vi "PH_Synchrolock_Watch.Investigeate Trace.vi"(0 "Threshold":dbl, 1 "Width":i32, 2 "X Increment":dbl, 3 "Waveform Array":dbl[](array[numeric]), 5 "error in":errorcluster) -> (14 "Mean Amplitude":dbl, 15 "Peak Locations":dbl[](array[numeric]), 19 "error out":errorcluster)   [LabVIEW 2014, in "PH_Synchrolock_Watch.lvlib"]
doc: "This VI scales the incoming waveform, detects the pek position(s) and further information."
uses:
  PH_Synchrolock_Watch.lvlib
  <vilib>/Analysis/baseanly.llb/Mean (DBL).vi
  <vilib>/measure/mamon.llb/Waveform Peak Detection for 1 Chan.vi
  <vilib>/measure/NI_MAPro.lvlib
  <vilib>/Analysis/NI_AALBase.lvlib
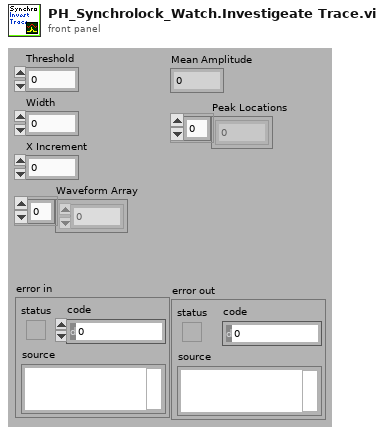
[diagram p1: front panel]
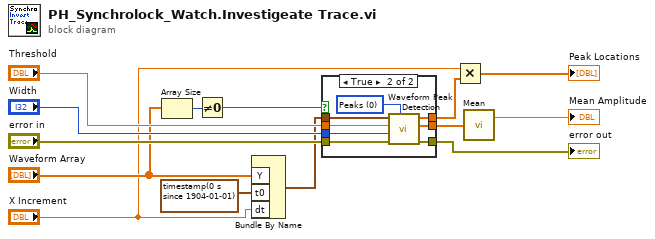
[diagram p0: block diagram]
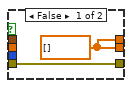
[diagram p2: hidden frame]
diagram:
  n1 = Array Size(array="Waveform Array") -> (size(s)=w9:i32)
  n2 = Not Equal To 0?(x=w9) -> (x != 0?=w8:bool)
  n3 = Bundle By Name("Y"="Waveform Array", "t0"=timestamp(0 s since 1904-01-01), "dt"="X Increment") -> (w7:waveform(dbl))  [unwired: 1 out]
  n4 = case shown="True" w8 {
    tunnel: "Threshold" -> [_ w24]
    tunnel: [w16 w23] -> w5
    tunnel: w7 -> [_ w22]
    tunnel: [w16 w21] -> w2
    tunnel: "Width" -> [_ w20]
    tunnel: "error in" -> [w15 w19]
    tunnel: [w15 w18] -> w14
    frame False {
      w16 = dbl[] [] ("Locations")
    }
    frame True {
      w17 = u16 0 items=["Peaks", "Valleys"] ("peaks/valleys")
      n5 = call-poly <vilib>:"Waveform Peak Detection.vi"("peaks/valleys"=w17, "error in"=w19, "width"=w20, "threshold"=w24, "Signal In"=w22) -> ("error out"=w18:errorcluster, "Amplitudes"=w21:dbl[], "Locations"=w23:dbl[])  [unwired: 2 in, 2 out]
    }
  }
  "error out" <- w14
  n6 = Multiply(x="X Increment", y=w5) -> (x*y=→"Peak Locations":dbl[])
  n7 = call-poly <vilib>:"Mean.vi"("X"=w2) -> ("mean"=→"Mean Amplitude":dbl)  [unwired: 1 out]
